vi "Get Current Timestamp.vi"() -> (2 "Timestamp":T1)   [LabVIEW 2024, in "Sift Client.lvlib"]
doc: "Returns the UNIX timestamp in the Sift compatible format (seconds and nanoseconds)."
uses:
  Sift Client.lvlib
  Private/Typedefs/Timestamp.ctl
  <vilib>/LabVIEW Open Source Project/Epoch Date & Time/epoch.UNIX/Epoch.UNIX.lvclass
  <vilib>/LabVIEW Open Source Project/Epoch Date & Time/Get Epoch Time.vi
panel:
  in  "Timestamp 2":T1
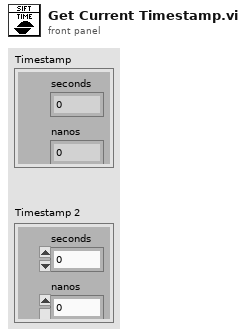
[diagram p1: front panel]
types:
  T1 = typedef "Sift Client.lvlib/Timestamp.ctl" = cluster{"seconds":i64, "nanos":i32}
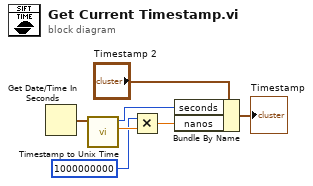
[diagram p0: block diagram]
diagram:
  n1 = Get Date/Time In Seconds() -> (seconds since 1Jan1904=w7:timestamp)
  n2 = call <vilib>:"Timestamp to Unix Time.vi"("Timestamp (now)"=w7) -> ("Fractional Second"=w6:dbl, "Unix Time (s)"=w4:i64)  [unwired: 9 in]
  n3 = Multiply(x=1000000000, y=w6) -> (x*y=w3:dbl)
  n4 = Bundle By Name(cluster="Timestamp 2", "seconds"=w4, "nanos"=w3) -> (→"Timestamp":T1)
